vi "LaunchDependency.vi"(6 "Shared Resource":bool, 8 "error in (no error)":errorcluster, 9 "Dependency Name":string, 10 "Dependency Type":refnum<class "SMO.lvclass">, 11 "SMO in":refnum<class "SMO.lvclass">) -> (0 "error out":errorcluster, 1 "Unique Name":string, 3 "SMO out":refnum<class "SMO.lvclass">)   [LabVIEW 2013, in "SMO.lvclass"]
uses:
  SMO.lvclass
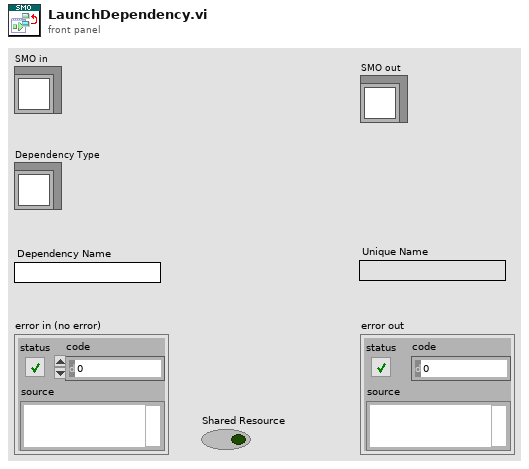
[diagram p1: front panel]
types:
  T1 = typedef "SMO.lvclass/SMOState --Enum.ctl" = enum16{"unknown", "Created", "Started", "Stopped"}
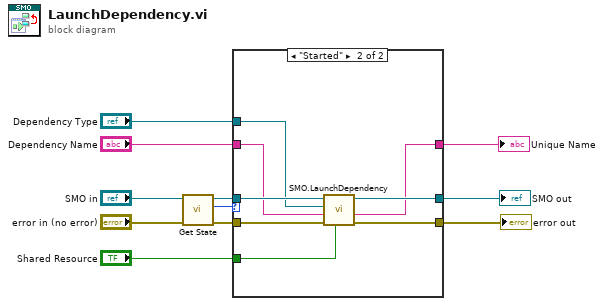
[diagram p0: block diagram]
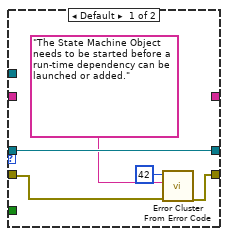
[diagram p2: hidden frame]
diagram:
  n1 = call "Get State.vi"("error in (no error)"="error in (no error)", "SMO"="SMO in") -> ("error out"=w8:errorcluster, "SMO State"=w5:T1, "SMO out"=w10:refnum<class "SMO.lvclass">)  [unwired: 7 in]
  n2 = case shown="\"Started\"" w5 {
    tunnel: w10 -> [w16 w24]
    tunnel: [w16 w23] -> w9
    tunnel: w8 -> [w14 w22]
    tunnel: [w15 w21] -> w6
    tunnel: "Dependency Type" -> [_ w20]
    tunnel: "Dependency Name" -> [_ w19]
    tunnel: [_ w18] -> w2
    tunnel: "Shared Resource" -> [_ w17]
    frame Default {
      n3 = call <vilib>:"Error Cluster From Error Code.vi"("error in (no error)"=w14, "error message (\"\")"="The State Machine Object needs to be started before a run-time dependency can be launched or added." ("error message (\"\")"), "error code (0)"=42) -> ("error out"=w15:errorcluster)  [unwired: 6 in]
    }
    frame "Started" {
      n4 = call "SMO.LaunchDependency.vi"("Shared Resource"=w17, "error in (no error)"=w22, "Dependency Name"=w19, "Dependency Type"=w20, "SMO in"=w24) -> ("error out"=w21:errorcluster, "Unique Name"=w18:string, "SMO out"=w23:refnum<class "SMO.lvclass">)  [unwired: 4 in]
    }
  }
  "error out" <- w6
  "SMO out" <- w9
  "Unique Name" <- w2
